vi "FGV Laser.vi"(8 "error in (no error)":errorcluster, 10 "FGV Laser Data In":T1, 11 "Action":T2=enum."Connect") -> (0 "error out":errorcluster, 3 "FGV Laser Data Out":T1)   [LabVIEW 2017]
uses:
  Action Laser.ctl
  FGV Laser Data.ctl
  <vilib>/Instr/_visa.llb/VISA Configure Serial Port (Instr).vi
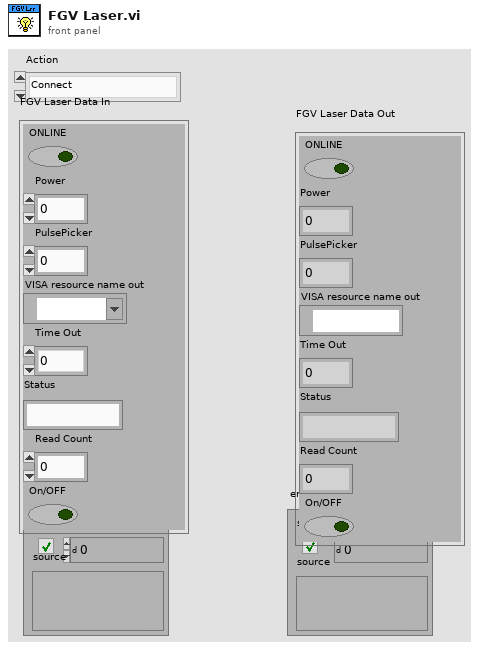
[diagram p1: front panel]
types:
  T1 = typedef "FGV Laser Data.ctl" = cluster{"ONLINE":bool, "Power":dbl, "PulsePicker":dbl, "VISA resource name out":refnum<visa-resource-name>, "Time Out":dbl, "Status":string, "Read Count":u32, "On/OFF":bool}
  T2 = typedef "Action Laser.ctl" = enum16{"Initialize", "Connect", "Disconnect", "Set Power", "Get Power", "Set Pulse Picker", "Get Pulse Picker", "Laser ON", "Laser OFF", "Read Visa"}
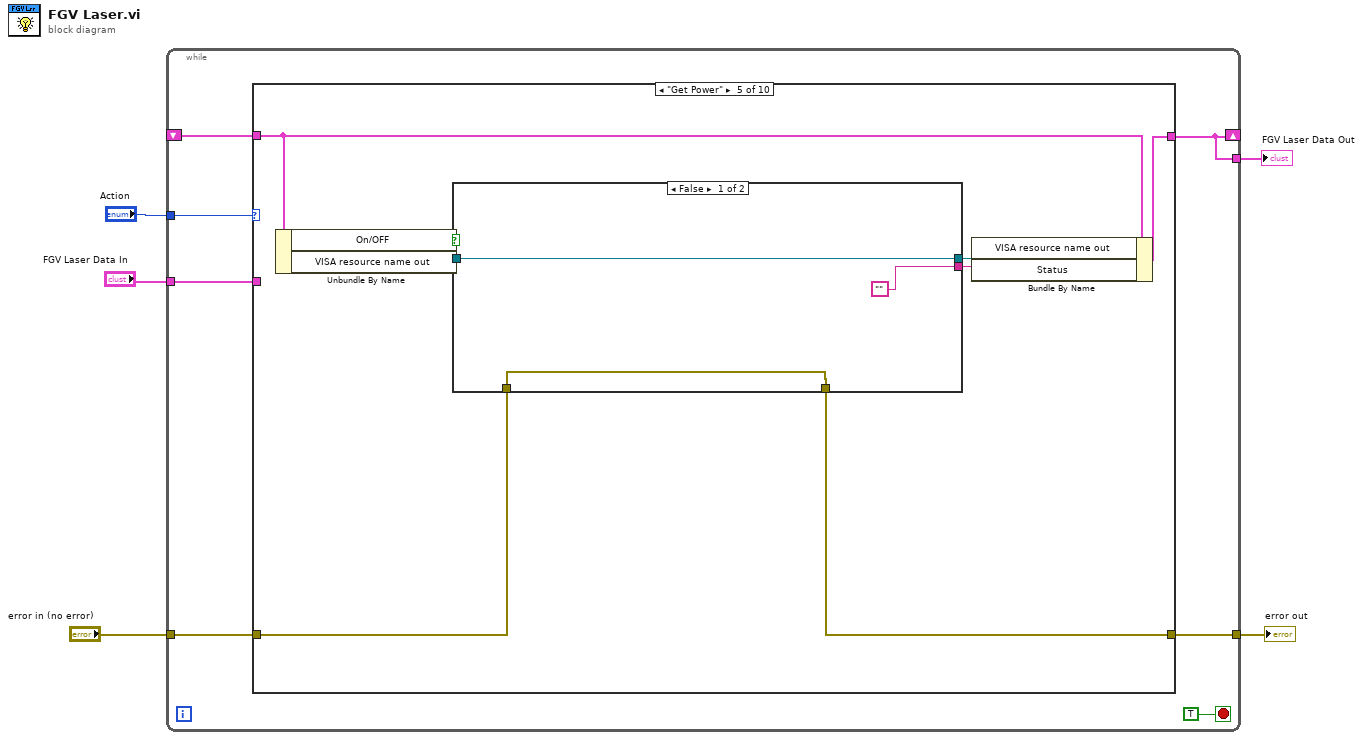
[diagram p0: block diagram]
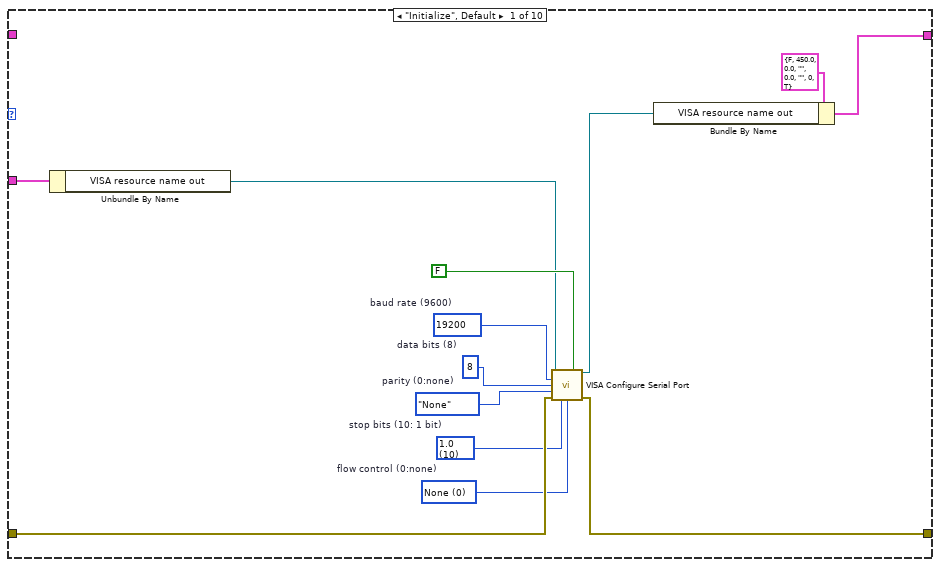
[diagram p2: hidden frame]
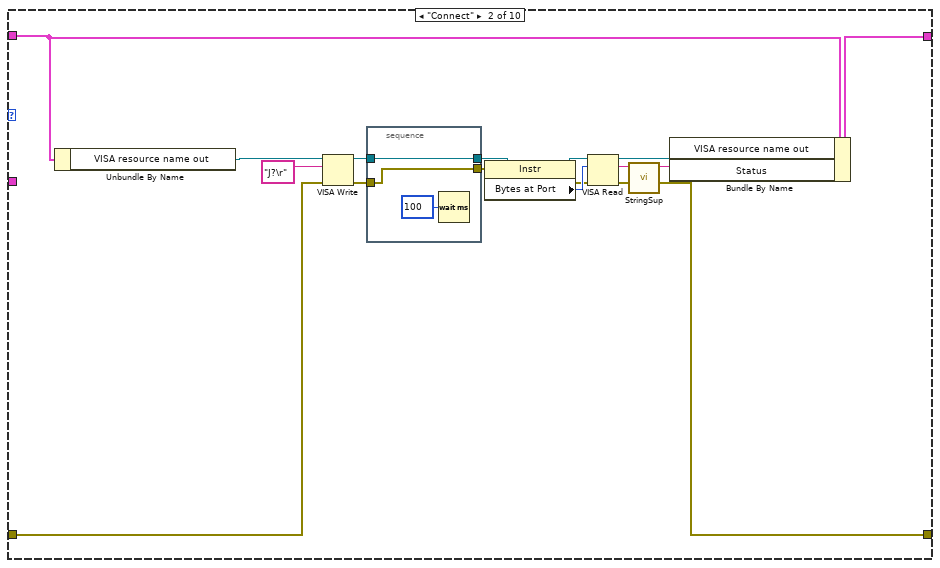
[diagram p3: hidden frame]
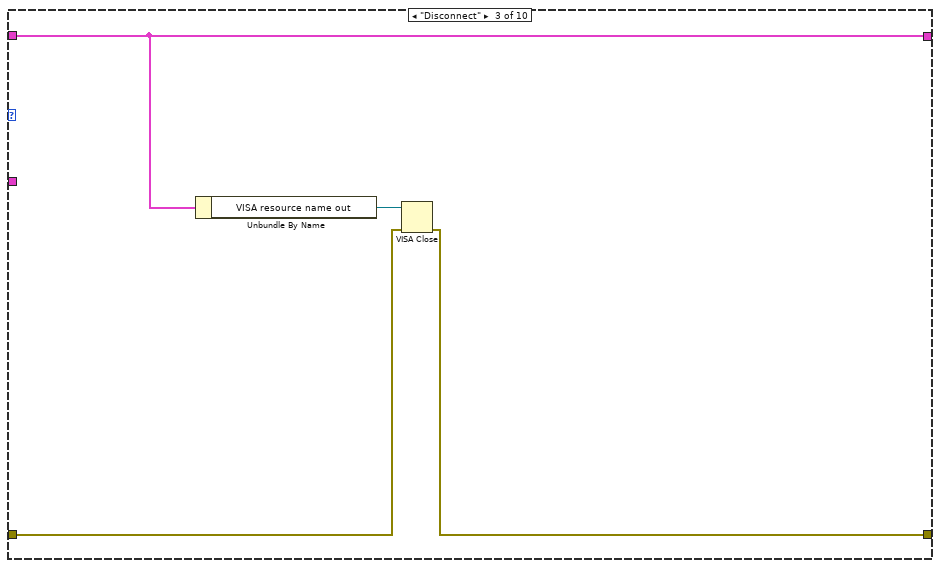
[diagram p4: hidden frame]
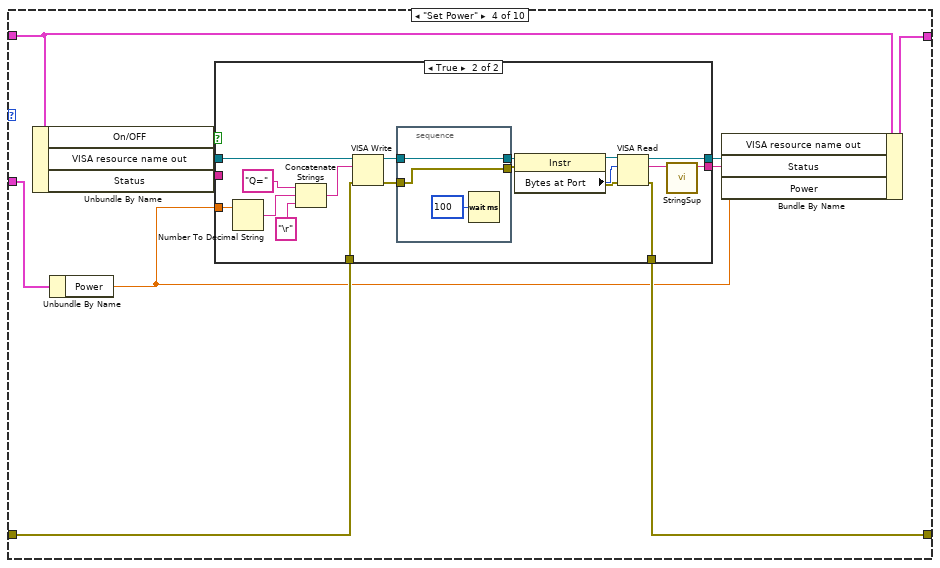
[diagram p5: hidden frame]
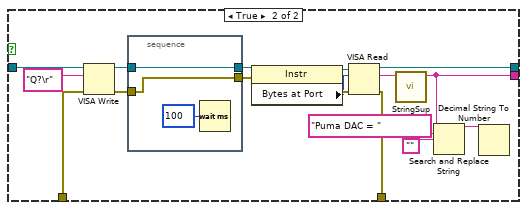
[diagram p7: hidden frame]
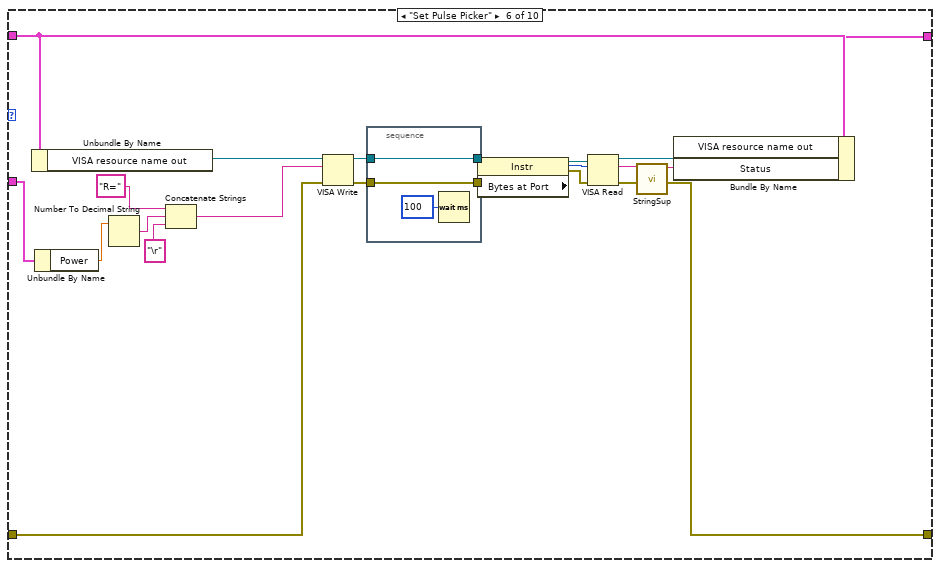
[diagram p8: hidden frame]
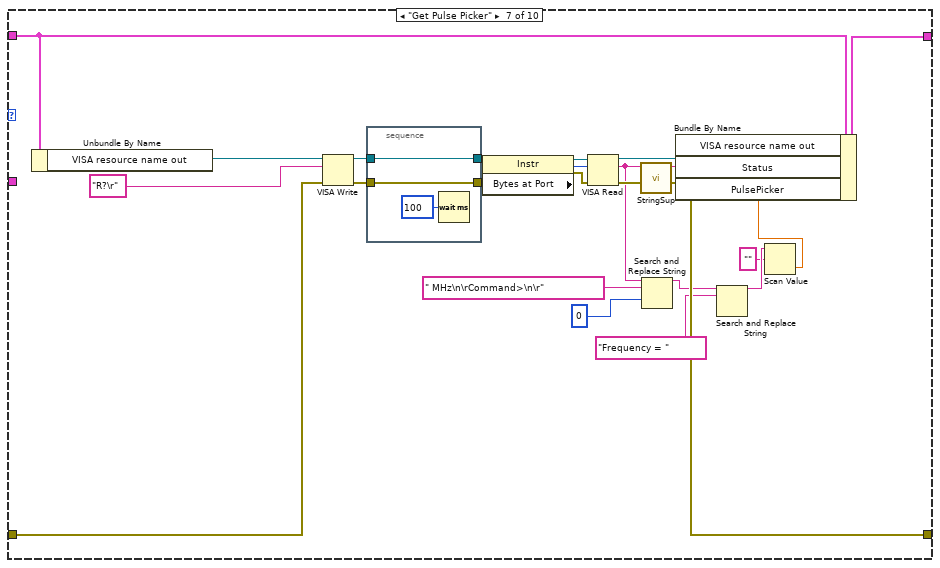
[diagram p9: hidden frame]
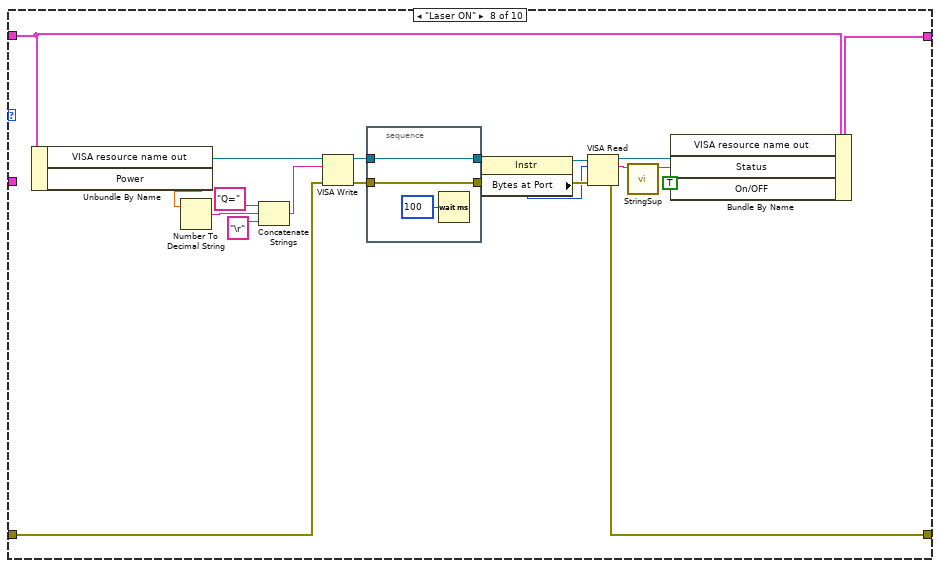
[diagram p10: hidden frame]
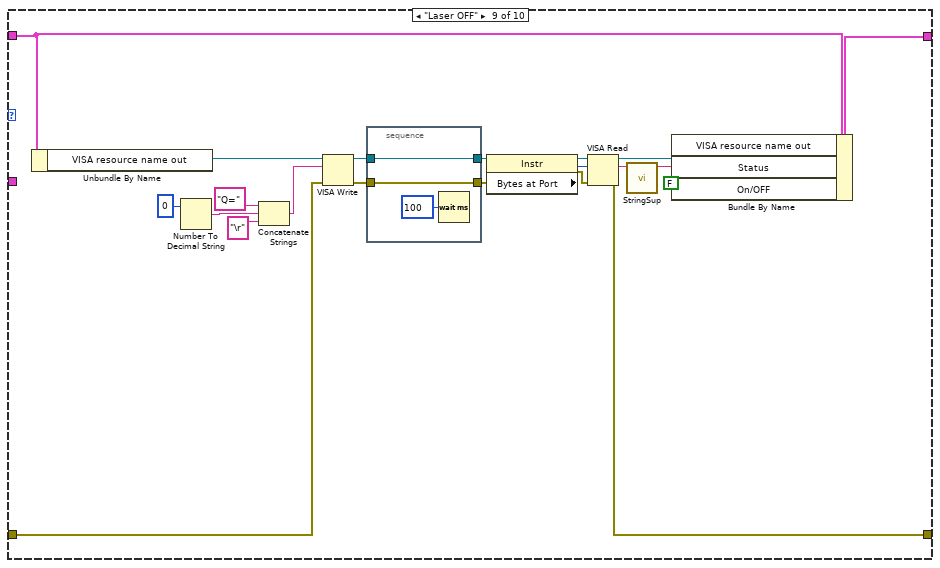
[diagram p11: hidden frame]
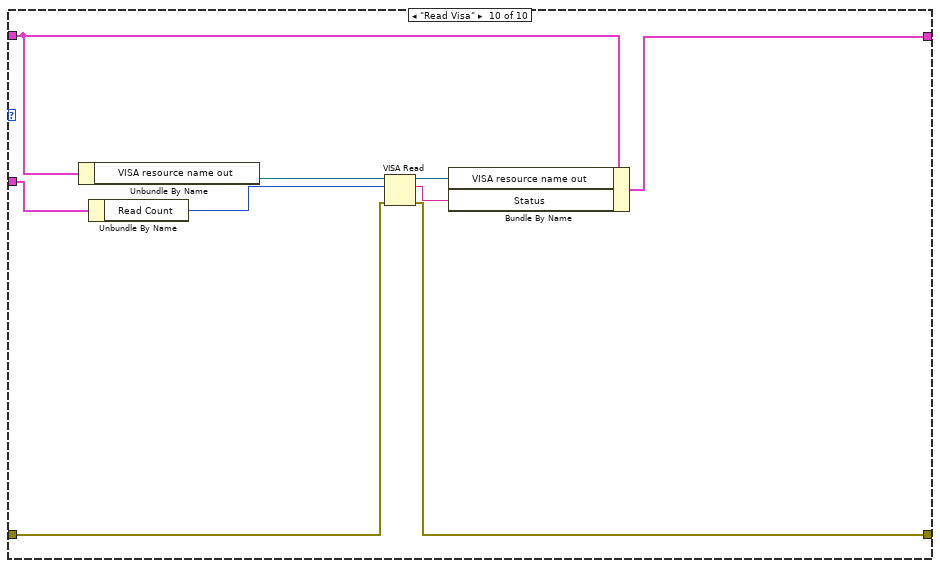
[diagram p12: hidden frame]
diagram:
  n1 = while {
    tunnel: "Action" -> [w11]
    tunnel: "error in (no error)" -> [w10]
    tunnel: [w9] -> w3
    shift-right: [w6] -> _
    shift-left: _ -> [w8]
    tunnel: "FGV Laser Data In" -> [w7]
    tunnel: [w6] -> w1
    stop <- TRUE stop-if-true
    n2 = case shown="\"Get Power\"" w11 {
      tunnel: [w22 w33 w45 w54 w86 w128 w154 w178 w202 w219] -> w9
      tunnel: w10 -> [w23 w40 w46 w58 w90 w134 w160 w184 w208 w220]
      tunnel: [w19 w37 w48 w56 w88 w132 w158 w182 w206 w213] -> w6
      tunnel: w8 -> [_ w38 w48 w57 w89 w133 w159 w183 w207 w216]
      tunnel: w7 -> [w21 _ _ w53 _ w127 _ _ _ w218]
      frame "Initialize", Default {
        w15 = u16 0 items=["None", "XON/XOFF", "RTS/CTS", "XON/XOFF & RTS/CTS", "DTR/DSR", "XON/XOFF & DTR/DSR"]  # flow control (0:none)
        w16 = u16 10 items=["1.0"=10, "1.5"=15, "2.0"=20]  # stop bits (10: 1 bit)
        w17 = enum16{"None", "Odd", "Even", "Mark", "Space"}."None"  # parity (0:none)
        w24 = u16 8  # data bits (8)
        w25 = u32 19200  # baud rate (9600)
        n3 = Unbundle By Name(w21) -> ("VISA resource name out"=w13:refnum<visa-resource-name>)
        n4 = call-poly "VISA Configure Serial Port"("VISA resource name"=w13, "Enable Termination\nChar (T)"=FALSE ("Enable Termination\nChar (T)"), "baud rate (9600)"=w25, "data bits (8)"=w24, "parity (0:none)"=w17, "error in (no error)"=w23, "stop bits (10: 1 bit)"=w16, "flow control (0:none)"=w15) -> ("VISA resource name out"=w18:refnum<visa-resource-name>, "error out"=w22:errorcluster)  [unwired: 6 in]
        n5 = Bundle By Name(cluster=T1 {"ONLINE"=FALSE, "Power"=450.0, "PulsePicker"=0.0, "VISA resource name out"="", "Time Out"=0.0, "Status"="", "Read Count"=0, "On/OFF"=TRUE} ("FGV Laser Data"), "VISA resource name out"=w18) -> (w19:T1)
      }
      frame "Connect" {
        n6 = Unbundle By Name(w38) -> ("VISA resource name out"=w41:refnum<visa-resource-name>)
        n7 = VISA Write(VISA resource name=w41, write buffer="J?\r", error in (no error)=w40) -> (VISA resource name out=w35:refnum<visa-resource-name>, error out=w36:errorcluster)  [unwired: 1 out]
        n8 = stacked-sequence {
          tunnel: w36 -> [w42]
          tunnel: w35 -> [w43]
          tunnel: [w43] -> w32
          tunnel: [w42] -> w29
          frame #0 {
            n9 = Wait (ms)(milliseconds to wait=u32 100) -> ()  [unwired: 1 out]
          }
        }
        n10 = property class="Instr"(reference=w32, error in=w29) -> (reference out=w30:refnum<visa-resource-name>, error out=w28:errorcluster, "Bytes at Port"=w31:u32)
        n11 = VISA Read(VISA resource name=w30, byte count=w31, error in (no error)=w28) -> (VISA resource name out=w34:refnum<visa-resource-name>, read buffer=w27:string, error out=w33:errorcluster)  [unwired: 1 out]
        n12 = call "StringSup.vi"("String"=w27) -> ("result string"=w26:string)  [unwired: 10 in]
        n13 = Bundle By Name(cluster=w38, "VISA resource name out"=w34, "Status"=w26) -> (w37:T1)
      }
      frame "Disconnect" {
        n14 = Unbundle By Name(w48) -> ("VISA resource name out"=w47:refnum<visa-resource-name>)
        n15 = VISA Close(VISA resource name=w47, error in (no error)=w46) -> (error out=w45:errorcluster)
      }
      frame "Set Power" {
        n16 = Unbundle By Name(w57) -> ("On/OFF"=w50:bool, "VISA resource name out"=w59:refnum<visa-resource-name>, "Status"=w49:string)
        n17 = Unbundle By Name(w53) -> ("Power"=w52:dbl)
        n18 = case shown="True" w50 {
          tunnel: w59 -> [w61 w80]
          tunnel: w58 -> [w60 w79]
          tunnel: [w61 w76] -> w55
          tunnel: [w60 w75] -> w54
          tunnel: w52 -> [_ w70]
          tunnel: [w62 w63] -> w51
          tunnel: w49 -> [w62 _]
          frame False {
          }
          frame True {
            n19 = Number To Decimal String(number=w70) -> (decimal integer string=w73:string)  [unwired: 1 in]
            n20 = Concatenate Strings("Q=" ("write buffer"), w73, "\r" ("string")) -> (w71:string)
            n21 = VISA Write(VISA resource name=w80, write buffer=w71, error in (no error)=w79) -> (VISA resource name out=w77:refnum<visa-resource-name>, error out=w78:errorcluster)  [unwired: 1 out]
            n22 = stacked-sequence {
              tunnel: w78 -> [w81]
              tunnel: w77 -> [w82]
              tunnel: [w82] -> w69
              tunnel: [w81] -> w68
              frame #0 {
                n23 = Wait (ms)(milliseconds to wait=u32 100) -> ()  [unwired: 1 out]
              }
            }
            n24 = property class="Instr"(reference=w69, error in=w68) -> (reference out=w67:refnum<visa-resource-name>, error out=w65:errorcluster, "Bytes at Port"=w66:u32)
            n25 = VISA Read(VISA resource name=w67, byte count=w66, error in (no error)=w65) -> (VISA resource name out=w76:refnum<visa-resource-name>, read buffer=w64:string, error out=w75:errorcluster)  [unwired: 1 out]
            n26 = call "StringSup.vi"("String"=w64) -> ("result string"=w63:string)  [unwired: 10 in]
          }
        }
        n27 = Bundle By Name(cluster=w57, "VISA resource name out"=w55, "Status"=w51, "Power"=w52) -> (w56:T1)
      }
      frame "Get Power" {
        n28 = Unbundle By Name(w89) -> ("On/OFF"=w84:bool, "VISA resource name out"=w91:refnum<visa-resource-name>)
        n29 = case shown="False" w84 {
          tunnel: w91 -> [w94 w111]
          tunnel: w90 -> [w93 w110]
          tunnel: [w94 w107] -> w87
          tunnel: [w93 w106] -> w86
          tunnel: ["" w95] -> w85
          frame False {
          }
          frame True {
            n30 = VISA Write(VISA resource name=w111, write buffer="Q?\r", error in (no error)=w110) -> (VISA resource name out=w108:refnum<visa-resource-name>, error out=w109:errorcluster)  [unwired: 1 out]
            n31 = stacked-sequence {
              tunnel: w109 -> [w112]
              tunnel: w108 -> [w113]
              tunnel: [w113] -> w104
              tunnel: [w112] -> w103
              frame #0 {
                n32 = Wait (ms)(milliseconds to wait=u32 100) -> ()  [unwired: 1 out]
              }
            }
            n33 = property class="Instr"(reference=w104, error in=w103) -> (reference out=w102:refnum<visa-resource-name>, error out=w101:errorcluster, "Bytes at Port"=w100:u32)
            n34 = VISA Read(VISA resource name=w102, byte count=w100, error in (no error)=w101) -> (VISA resource name out=w107:refnum<visa-resource-name>, read buffer=w99:string, error out=w106:errorcluster)  [unwired: 1 out]
            n35 = call "StringSup.vi"("String"=w99) -> ("result string"=w95:string)  [unwired: 10 in]
            n36 = Search and Replace String(input string=w95, search string="Puma DAC = ", replace string="") -> (result string=w96:string)  [unwired: 5 in, 3 out]
            n37 = Decimal String To Number(string=w96) -> ()  [unwired: 2 in, 2 out]
          }
        }
        n38 = Bundle By Name(cluster=w89, "VISA resource name out"=w87, "Status"=w85) -> (w88:T1)
      }
      frame "Set Pulse Picker" {
        n39 = Unbundle By Name(w133) -> ("VISA resource name out"=w135:refnum<visa-resource-name>)
        n40 = Unbundle By Name(w127) -> ("Power"=w126:dbl)
        n41 = Number To Decimal String(number=w126) -> (decimal integer string=w124:string)  [unwired: 1 in]
        n42 = Concatenate Strings("R=" ("write buffer"), w124, "\r" ("string")) -> (w122:string)
        n43 = VISA Write(VISA resource name=w135, write buffer=w122, error in (no error)=w134) -> (VISA resource name out=w130:refnum<visa-resource-name>, error out=w131:errorcluster)  [unwired: 1 out]
        n44 = stacked-sequence {
          tunnel: w131 -> [w136]
          tunnel: w130 -> [w137]
          tunnel: [w137] -> w121
          tunnel: [w136] -> w120
          frame #0 {
            n45 = Wait (ms)(milliseconds to wait=u32 100) -> ()  [unwired: 1 out]
          }
        }
        n46 = property class="Instr"(reference=w121, error in=w120) -> (reference out=w119:refnum<visa-resource-name>, error out=w118:errorcluster, "Bytes at Port"=w117:u32)
        n47 = VISA Read(VISA resource name=w119, byte count=w117, error in (no error)=w118) -> (VISA resource name out=w129:refnum<visa-resource-name>, read buffer=w116:string, error out=w128:errorcluster)  [unwired: 1 out]
        n48 = call "StringSup.vi"("String"=w116) -> ("result string"=w115:string)  [unwired: 10 in]
        n49 = Bundle By Name(cluster=w133, "VISA resource name out"=w129, "Status"=w115) -> (w132:T1)
      }
      frame "Get Pulse Picker" {
        n50 = Unbundle By Name(w159) -> ("VISA resource name out"=w161:refnum<visa-resource-name>)
        n51 = VISA Write(VISA resource name=w161, write buffer="R?\r", error in (no error)=w160) -> (VISA resource name out=w156:refnum<visa-resource-name>, error out=w157:errorcluster)  [unwired: 1 out]
        n52 = stacked-sequence {
          tunnel: w157 -> [w162]
          tunnel: w156 -> [w163]
          tunnel: [w163] -> w145
          tunnel: [w162] -> w144
          frame #0 {
            n53 = Wait (ms)(milliseconds to wait=u32 100) -> ()  [unwired: 1 out]
          }
        }
        n54 = property class="Instr"(reference=w145, error in=w144) -> (reference out=w143:refnum<visa-resource-name>, error out=w141:errorcluster, "Bytes at Port"=w142:u32)
        n55 = VISA Read(VISA resource name=w143, byte count=w142, error in (no error)=w141) -> (VISA resource name out=w155:refnum<visa-resource-name>, read buffer=w140:string, error out=w154:errorcluster)  [unwired: 1 out]
        n56 = call "StringSup.vi"("String"=w140) -> ("result string"=w139:string)  [unwired: 10 in]
        n57 = Search and Replace String(input string=w140, search string=" MHz\n\rCommand>\n\r" ("substring (\"\")"), offset=0 ("offset (0)")) -> (result string=w151:string)  [unwired: 5 in, 3 out]
        n58 = Search and Replace String(input string=w151, search string="Frequency = ") -> (result string=w148:string)  [unwired: 6 in, 3 out]
        n59 = Scan Value(string=w148, format string="") -> (value=w146:dbl)  [unwired: 1 in, 1 out]
        n60 = Bundle By Name(cluster=w159, "VISA resource name out"=w155, "Status"=w139, "PulsePicker"=w146) -> (w158:T1)
      }
      frame "Laser ON" {
        n61 = Unbundle By Name(w183) -> ("VISA resource name out"=w185:refnum<visa-resource-name>, "Power"=w173:dbl)
        n62 = Number To Decimal String(number=w173) -> (decimal integer string=w176:string)  [unwired: 1 in]
        n63 = Concatenate Strings("Q=" ("write buffer"), w176, "\r" ("string")) -> (w174:string)
        n64 = VISA Write(VISA resource name=w185, write buffer=w174, error in (no error)=w184) -> (VISA resource name out=w180:refnum<visa-resource-name>, error out=w181:errorcluster)  [unwired: 1 out]
        n65 = stacked-sequence {
          tunnel: w181 -> [w186]
          tunnel: w180 -> [w187]
          tunnel: [w187] -> w172
          tunnel: [w186] -> w171
          frame #0 {
            n66 = Wait (ms)(milliseconds to wait=u32 100) -> ()  [unwired: 1 out]
          }
        }
        n67 = property class="Instr"(reference=w172, error in=w171) -> (reference out=w170:refnum<visa-resource-name>, error out=w169:errorcluster, "Bytes at Port"=w168:u32)
        n68 = VISA Read(VISA resource name=w170, byte count=w168, error in (no error)=w169) -> (VISA resource name out=w179:refnum<visa-resource-name>, read buffer=w167:string, error out=w178:errorcluster)  [unwired: 1 out]
        n69 = call "StringSup.vi"("String"=w167) -> ("result string"=w166:string)  [unwired: 10 in]
        n70 = Bundle By Name(cluster=w183, "VISA resource name out"=w179, "Status"=w166, "On/OFF"=TRUE) -> (w182:T1)
      }
      frame "Laser OFF" {
        n71 = Unbundle By Name(w207) -> ("VISA resource name out"=w209:refnum<visa-resource-name>)
        n72 = Number To Decimal String(number=0) -> (decimal integer string=w200:string)  [unwired: 1 in]
        n73 = Concatenate Strings("Q=" ("write buffer"), w200, "\r" ("string")) -> (w198:string)
        n74 = VISA Write(VISA resource name=w209, write buffer=w198, error in (no error)=w208) -> (VISA resource name out=w204:refnum<visa-resource-name>, error out=w205:errorcluster)  [unwired: 1 out]
        n75 = stacked-sequence {
          tunnel: w205 -> [w210]
          tunnel: w204 -> [w211]
          tunnel: [w211] -> w196
          tunnel: [w210] -> w195
          frame #0 {
            n76 = Wait (ms)(milliseconds to wait=u32 100) -> ()  [unwired: 1 out]
          }
        }
        n77 = property class="Instr"(reference=w196, error in=w195) -> (reference out=w194:refnum<visa-resource-name>, error out=w192:errorcluster, "Bytes at Port"=w193:u32)
        n78 = VISA Read(VISA resource name=w194, byte count=w193, error in (no error)=w192) -> (VISA resource name out=w203:refnum<visa-resource-name>, read buffer=w191:string, error out=w202:errorcluster)  [unwired: 1 out]
        n79 = call "StringSup.vi"("String"=w191) -> ("result string"=w190:string)  [unwired: 10 in]
        n80 = Bundle By Name(cluster=w207, "VISA resource name out"=w203, "Status"=w190, "On/OFF"=FALSE) -> (w206:T1)
      }
      frame "Read Visa" {
        n81 = Unbundle By Name(w216) -> ("VISA resource name out"=w221:refnum<visa-resource-name>)
        n82 = Unbundle By Name(w218) -> ("Read Count"=w217:u32)
        n83 = VISA Read(VISA resource name=w221, byte count=w217, error in (no error)=w220) -> (VISA resource name out=w215:refnum<visa-resource-name>, read buffer=w214:string, error out=w219:errorcluster)  [unwired: 1 out]
        n84 = Bundle By Name(cluster=w216, "VISA resource name out"=w215, "Status"=w214) -> (w213:T1)
      }
    }
  }
  "error out" <- w3
  "FGV Laser Data Out" <- w1
